vi "_MDPtr To DVR.vi"(1 "MDPtr":T1) -> (0 "MDPtr DVR":refnum<data-value>)   [LabVIEW 2017, in "MDPtr.lvlib"]
uses:
  MDPtr.lvlib
  MDPtr TypeDef/MDPtr DataFrame-Memory.ctl
  MDPtr TypeDef/MDPtr DataFrame-Common.ctl
  <vilib>/Utility/Data Type/Type Definitions/Data Type.ctl
  MDPtr TypeDef/MDPtr.ctl
  <vilib>/Utility/Data Type/NI_Data Type.lvlib
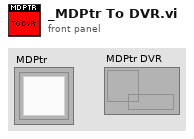
[diagram p1: front panel]
types:
  T1 = typedef "MDPtr.lvlib/MDPtr.ctl" = refnum<k1>
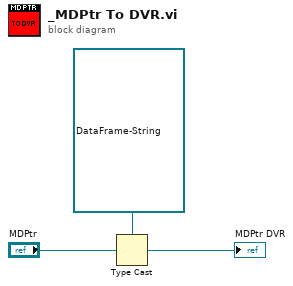
[diagram p0: block diagram]
diagram:
  n1 = Type Cast(type=refnum<data-value> refnum ("MDPtr DVR"), x="MDPtr") -> (*(type *) &x=→"MDPtr DVR":refnum<data-value>)
